vi "DownSampleData_82.vi"(8 "error in (no error)":errorcluster, 10 "Desired Sampling Rate":dbl=2000.0, 11 "Oversampled Values":waveform(sgl)[](array[waveform])) -> (0 "error out":errorcluster, 3 "Downsampled Data":waveform(sgl)[](array[waveform]))   [LabVIEW 2020]
doc: "This VI takes oversampled data and averages the data to downsample to the desired sampling rate. For instance, if data is captured at 2000 Hz for 1 second and the desired sampling rate is 50 Hz, every new data point is the result of averaging 40 data points (from the 2000 Hz data stream)."
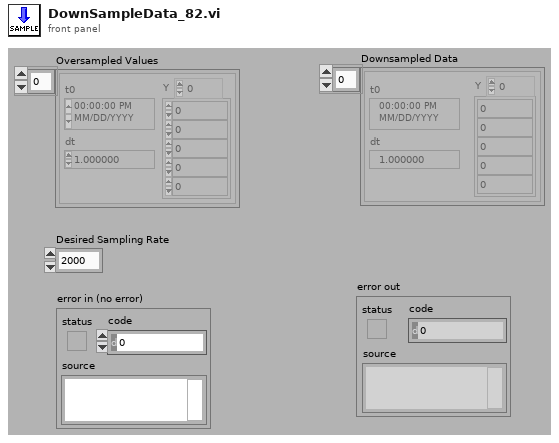
[diagram p1: front panel]
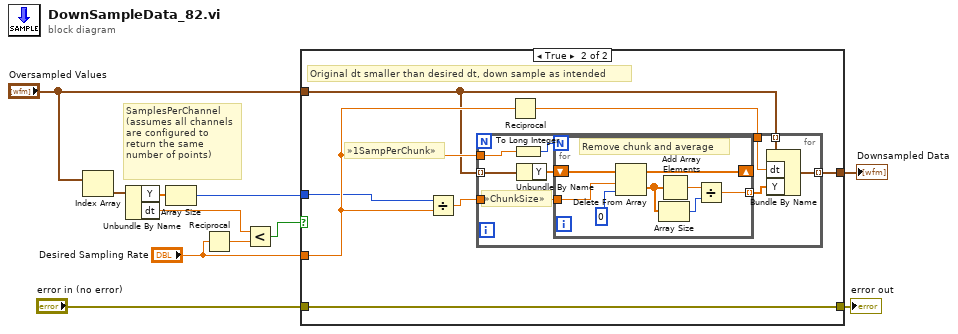
[diagram p0: block diagram]
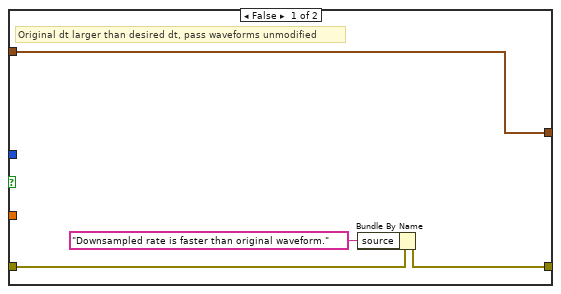
[diagram p2: hidden frame]
diagram:
  # "SamplesPerChannel\n(assumes all channels\nare configured to \nreturn the same \nnumber of points)"
  n1 = Index Array(array="Oversampled Values") -> (element=w9:waveform(sgl))  [unwired: 1 in]
  n2 = Unbundle By Name(w9) -> ("Y"=w8:sgl[], "dt"=w2:dbl)
  n3 = Array Size(array=w8) -> (size(s)=w7:i32)
  n4 = Reciprocal(x="Desired Sampling Rate") -> (1/x=w3:dbl)
  n5 = Less?(x=w2, y=w3) -> (x < y?=w1:bool)
  n6 = case shown="True" w1 {
    tunnel: "Desired Sampling Rate" -> [_ w21]
    tunnel: [w15 w19] -> w11
    tunnel: "Oversampled Values" -> [w15 w18]
    tunnel: w7 -> [_ w17]
    tunnel: [w13 w16] -> w6
    tunnel: "error in (no error)" -> [w14 w16]
    frame False {
      # "Original dt larger than desired dt, pass waveforms unmodified"
      n7 = Bundle By Name(cluster=w14, "source"="Downsampled rate is faster than original waveform.") -> (w13:errorcluster)
    }
    frame True {
      # "Original dt smaller than desired dt, down sample as intended"
      # "»1SampPerChunk»"
      n8 = Divide(x=w17, y=w21) -> (x/y=w22:dbl)
      n9 = Reciprocal(x=w21) -> (1/x=w20:dbl)
      n10 = for {
        tunnel: w18 -> [w31] mode=indexing
        tunnel: [w25] -> w19 mode=indexing
        tunnel: w21 -> [w29]
        tunnel: w22 -> [w28]
        tunnel: w20 -> [w26]
        tunnel: w18 -> [w24] mode=indexing
        # "»ChunkSize»"
        n11 = To Long Integer(number=w29) -> (32bit integer=w23:i32)
        n12 = Unbundle By Name(w31) -> ("Y"=w30:sgl[])
        n13 = for {
          N: w23 -> [_]
          tunnel: [w39] -> w27 mode=indexing
          shift-right: [w35] -> _
          shift-left: w30 -> [w36]
          tunnel: w28 -> [w34]
          # "Remove chunk and average"
          n14 = Delete From Array(array=w36, length=w34, index=0) -> (deleted portion=w33:sgl[], array with subset deleted=w35:sgl[])
          n15 = Array Size(array=w33) -> (size(s)=w32:i32)
          n16 = Add Array Elements(numeric array=w33) -> (sum=w38:sgl)
          n17 = Divide(x=w38, y=w32) -> (x/y=w39:sgl)
        }
        n18 = Bundle By Name(cluster=w24, "dt"=w26, "Y"=w27) -> (w25:waveform(sgl))
      }
    }
  }
  "Downsampled Data" <- w11
  "error out" <- w6
